vi "Get associated LabVIEW error.vi"(11 "SubscribeResult JSON in":refnum<class "SubscribeResult JSON.lvclass">) -> (2 "LabVIEW Equivalent Error":errorcluster, 3 "SubscribeResult JSON out":refnum<class "SubscribeResult JSON.lvclass">)   [LabVIEW 2020, in "wamplv.lvlib" / "SubscribeResult JSON.lvclass"]
uses:
  SubscribeResult JSON.lvclass
  SubscribeResult JSON.lvclass/SubscribeResult JSON.ctl
  Private/Message loop classes/ErrorOrSuccess JSON/ErrorOrSuccess JSON.lvclass
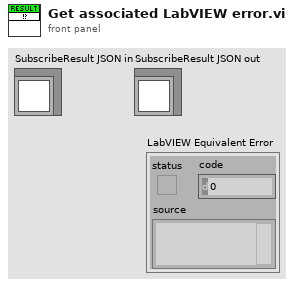
[diagram p1: front panel]
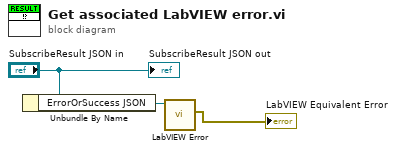
[diagram p0: block diagram]
diagram:
  n1 = Unbundle By Name("SubscribeResult JSON in") -> ("ErrorOrSuccess JSON"=w2:refnum<class "ErrorOrSuccess JSON.lvclass">)
  n2 = call-dynamic "LabVIEW Error.vi"("ErrorOrSuccess JSON in"=w2) -> ("Associated LabVIEW Error"=→"LabVIEW Equivalent Error":errorcluster)  [unwired: 9 in, 1 out]
  "SubscribeResult JSON out" <- "SubscribeResult JSON in"
